vi "Large current measurement readings.vi"() -> ()   [LabVIEW 2016, in "Top Level.lvlib"]
doc: "This vi displays current measurements in a large format"
uses:
  Top Level.lvlib
  cRIO code/SCA/controls/Vertical Rod states.ctl
  Features/features/features.lvlib
  sub-VIs/sub-VIs.lvlib
panel:
  in  "Tab Control":enum32{"measurements", "error and scale factor"}(tab)
  out "Sample Rod status":T1
  in  "rare count rate or stable":bool
  out "injector current":dbl format="%.2p"
  out "Current measurements":dbl(graph)
  out "offset cup Actual":dbl format="%#_5g"
  out "Current":dbl format="%#_4p"
  in  "stop":bool
  in  "error in (no error)":errorcluster
  out "error out":errorcluster
  out "Numeric":i32
  # "Rare count rate"
  # "Stable current"
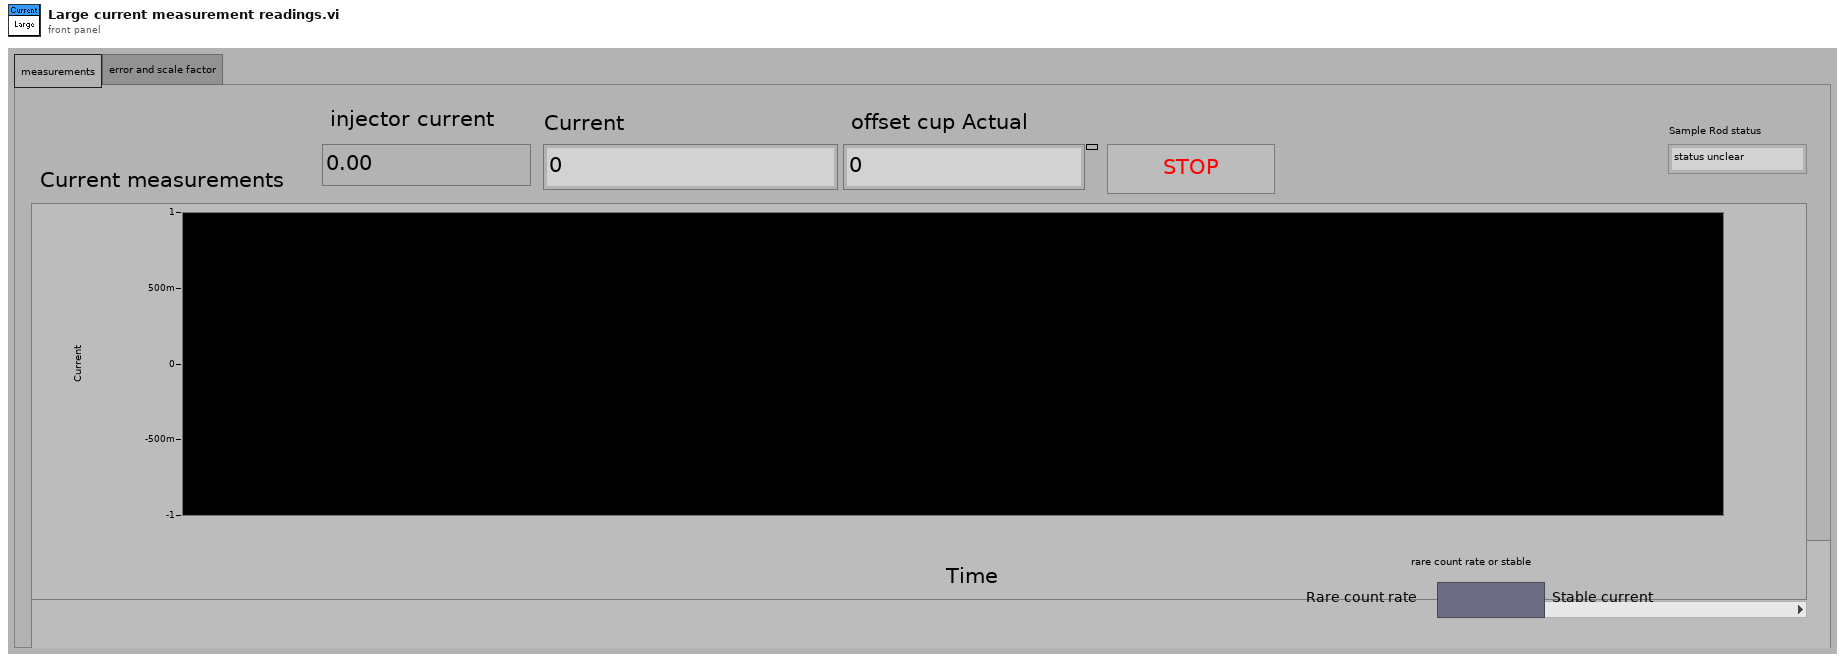
[diagram p1: front panel]
types:
  T1 = typedef "Vertical Rod states.ctl" = enum16{"status unclear", "rod down", "rod up"}
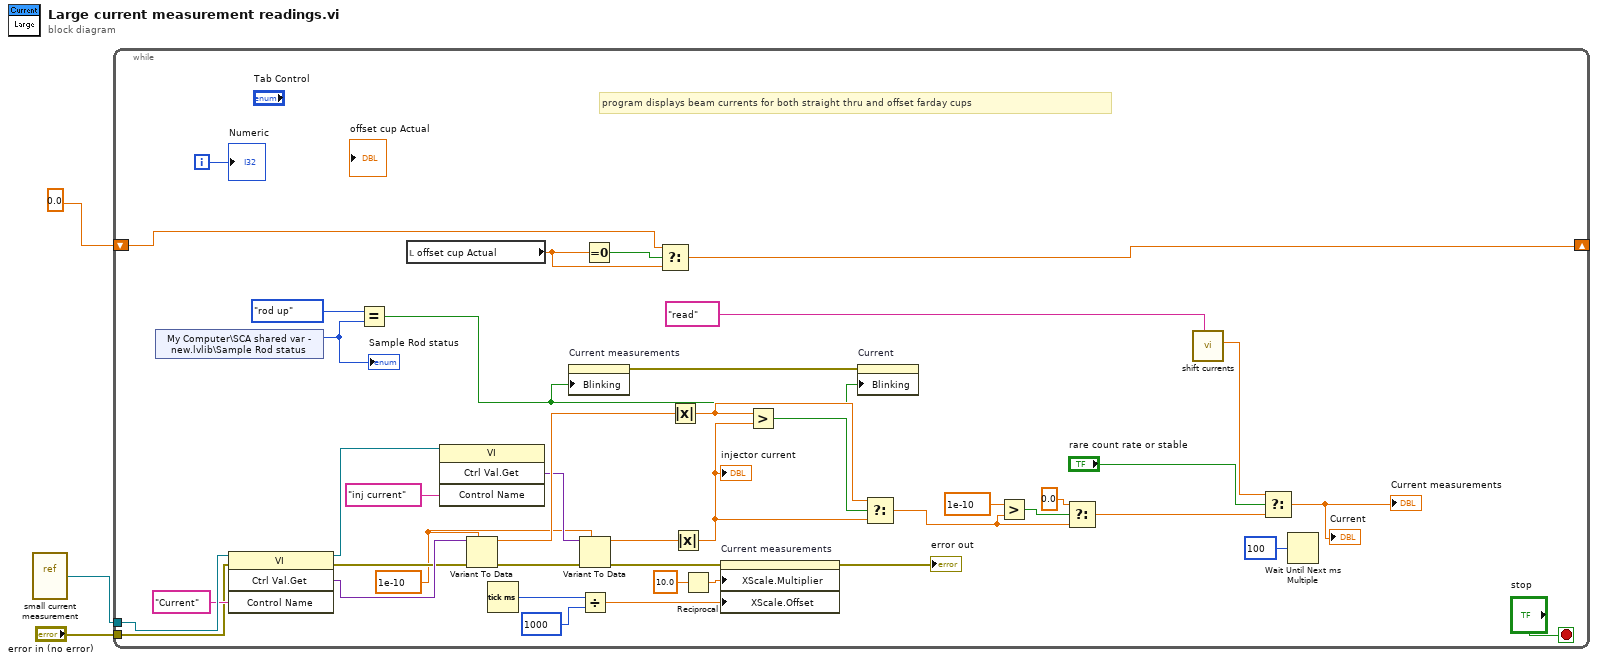
[diagram p0: block diagram]
diagram:
  n1 = vi-ref "small current measurement.vi"() -> (w2:refnum<vi>)
  n2 = while {
    shift-right: [w37] -> _
    shift-left: 0.0 -> [w38]
    tunnel: "error in (no error)" -> [w33]
    tunnel: w2 -> [w35]
    i -> [w30]
    stop <- "stop" stop-if-true
    w18 = 1e-10 ("x")
    # "program displays beam currents for both straight thru and offset farday cups"
    n3 = shared-variable "My Computer\\SCA shared var - new.lvlib\\Sample Rod status"() -> (w6:T1)  [unwired: 1 in, 1 out]
    "Sample Rod status" <- w6
    n4 = invoke class="VI" method="Ctrl Val.Get"(reference=w35, error in=w33, "Control Name"="Current") -> (reference out=w21:refnum<vi>, error out=w28:errorcluster, "Get Control Value Variant"=w32:variant)  [unwired: 1 in, 1 out]
    n5 = Equal?(x=Vertical_Rod_states."rod up", y=w6) -> (x = y?=w4:bool)
    n6 = local read "offset cup Actual"() -> (w29:dbl)
    n7 = invoke class="VI" method="Ctrl Val.Get"(reference=w21, "Control Name"="inj current") -> ("Get Control Value Variant"=w19:variant)  [unwired: 2 in, 3 out]
    n8 = Variant To Data(error in=w28, type=w18, Variant=w32) -> (data=w31:dbl, error out=w17:errorcluster)
    n9 = Tick Count (ms)() -> (millisecond timer value=w7:u32)
    n10 = property on="Current measurements" class="WFChart (strict)"("Blinking"=w4) -> (error out=w22:errorcluster)  [unwired: 2 in, 1 out]
    n11 = Variant To Data(error in=w17, type=w18, Variant=w19) -> (data=w16:dbl, error out=w11:errorcluster)
    n12 = Divide(x=w7, y=u32 1000 ("x")) -> (x/y=w9:dbl)
    n13 = Equal To 0?(x=w29) -> (x = 0?=w39:bool)
    n14 = Select(t=w38, s=w39, f=w29) -> (s? t:f=w37:dbl)
    n15 = Absolute Value(x=w31) -> (abs(x)=w36:dbl)
    n16 = Absolute Value(x=w16) -> (abs(x)=w15:dbl)
    "injector current" <- w15
    n17 = Reciprocal(x=10.0) -> (1/x=w13:dbl)
    n18 = property on="Current measurements" class="WFChart (strict)"(error in=w11, "XScale.Multiplier"=w13, "XScale.Offset"=w9) -> (error out=→"error out":errorcluster)  [unwired: 1 in, 1 out]
    n19 = Greater?(x=w36, y=w15) -> (0:w40:bool)
    n20 = property on="Current" class="DigNum (strict)"(error in=w22, "Blinking"=w4) -> ()  [unwired: 1 in, 2 out]
    n21 = Select(t=w36, s=w40, f=w15) -> (s? t:f=w26:dbl)
    n22 = Greater?(x=1e-10, y=w26) -> (0:w42:bool)
    n23 = Select(t=0.0, s=w42, f=w26) -> (s? t:f=w23:dbl)
    n24 = call "shift currents.vi"("Combo Box"="read") -> ("current out"=w24:dbl)  [unwired: 10 in]
    n25 = Select(t=w24, s="rare count rate or stable", f=w23) -> (s? t:f=→"Current" →"Current measurements":dbl)
    n26 = Wait Until Next ms Multiple(millisecond multiple=u32 100) -> ()  [unwired: 1 out]
    "Numeric" <- w30
  }
